vi "Is FIFO Queue Name.vi"(11 "Name":string) -> (3 "FIFO Queue":bool)   [LabVIEW 2015, in "NI_AWS_SQS.lvlib" / "Queue.lvclass"]
uses:
  Queue.lvclass
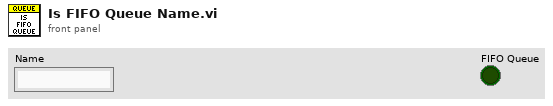
[diagram p1: front panel]
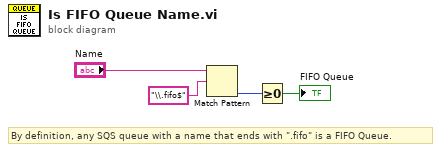
[diagram p0: block diagram]
diagram:
  # "By definition, any SQS queue with a name that ends with \".fifo\" is a FIFO Queue."
  n1 = Match Pattern(string="Name", regular expression="\\.fifo$") -> (offset past match=w2:i32)  [unwired: 1 in, 3 out]
  n2 = Greater Or Equal To 0?(x=w2) -> (x >= 0?=→"FIFO Queue":bool)
